vi "Test Create Folder and File.vi"   [LabVIEW 2018]
panel:
  # "See block diagram."
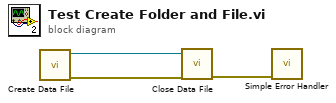
[diagram p0: block diagram]
diagram:
  n1 = call "Create Data File.vi"() -> ("Error Out"=w3:errorcluster, "File Refnum"=w1:refnum<file>)  [unwired: 10 in]
  n2 = call "Close Data File.vi"("error in"=w3, "File Refnum In"=w1) -> ("error out"=w2:errorcluster)  [unwired: 9 in]
  n3 = call <vilib>:"Simple Error Handler.vi"("error in (no error)"=w2) -> ()  [unwired: 4 in, 5 out]
